vi "BPSK_Channel.vi"(8 "error in (no error)":errorcluster caption="错误输入（无错误）", 9 "snr":i32, 10 "txSig":dbl[](array[numeric]) format="%#_13g", 11 "PathIn":path) -> (0 "error out":errorcluster caption="错误输出", 2 "rxSig":dbl[](array[numeric]), 3 "PathOut":path)   [LabVIEW 2015]
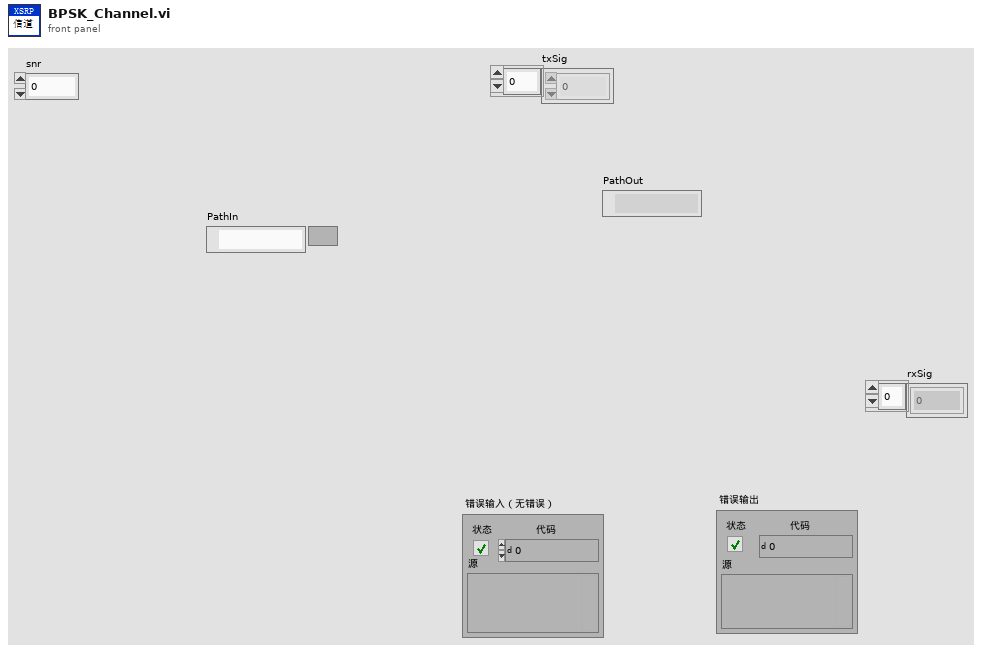
[diagram p1: front panel]
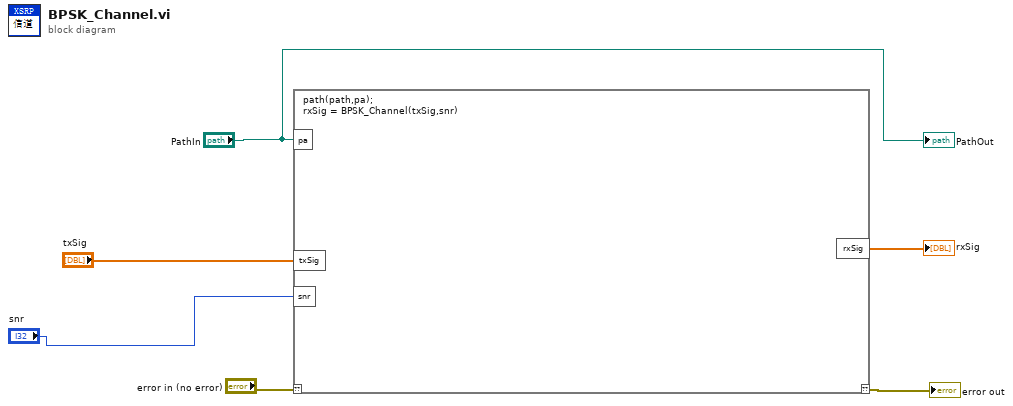
[diagram p0: block diagram]
diagram:
  n1 = script code="path(path,pa);\nrxSig = BPSK_Channel(txSig,snr)"("??"="error in (no error)", "pa"="PathIn", "txSig"="txSig", "snr"="snr") -> ("??"=→"error out":errorcluster, "rxSig"=→"rxSig":dbl[])
  "PathOut" <- "PathIn"
